vi "Read Roles.vi"(8 "error in (no error)":errorcluster, 11 "EnemyPossessionAtOurFieldPlay in":refnum<class "EnemyPossessionAtOurFieldPlay.lvclass">) -> (0 "error out":errorcluster, 2 "Roles":T1, 3 "EnemyPossessionAtOurFieldPlay out":refnum<class "EnemyPossessionAtOurFieldPlay.lvclass">)   [LabVIEW 2020, in "EnemyPossessionAtOurFieldPlay.lvclass"]
uses:
  EnemyPossessionAtOurFieldPlay.lvclass
  EnemyPossessionAtOurFieldRoles.ctl
  ShootRole_class/ShootRole.lvclass
  MarkerRole_class/MarkerRole.lvclass
  EnemyPossessionAtOurFieldPlay.lvclass/EnemyPossessionAtOurFieldPlay.ctl
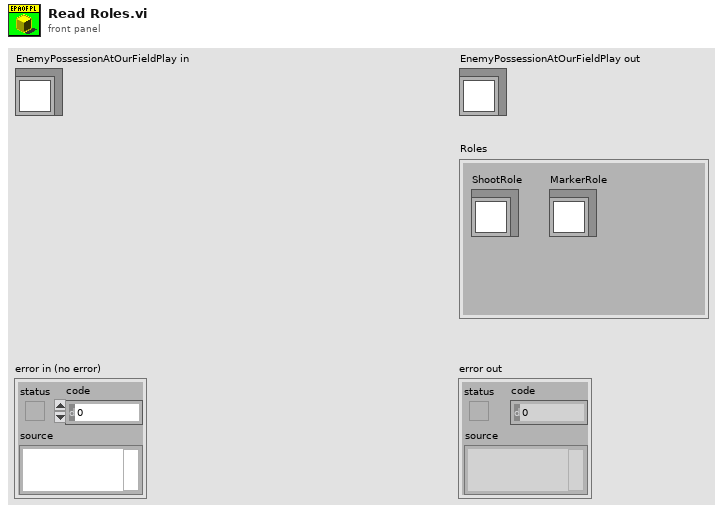
[diagram p1: front panel]
types:
  T1 = typedef "EnemyPossessionAtOurFieldRoles.ctl" = cluster{"ShootRole":refnum<class "ShootRole.lvclass">, "MarkerRole":refnum<class "MarkerRole.lvclass">}
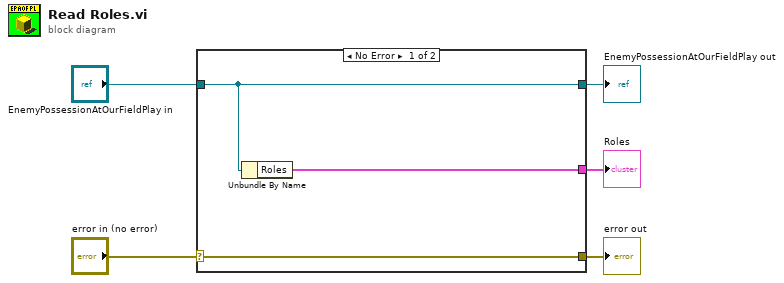
[diagram p0: block diagram]
diagram:
  n1 = case shown="No Error" "error in (no error)" {
    selector: "error in (no error)" -> [w8 w9]
    tunnel: [w8 w9] -> w4
    tunnel: [w7 w10] -> w2
    tunnel: "EnemyPossessionAtOurFieldPlay in" -> [w7 w10]
    tunnel: [w6 _] -> w1
    frame No Error {
      n2 = Unbundle By Name(w7) -> ("Roles"=w6:T1)
    }
    frame Error {
    }
  }
  "error out" <- w4
  "EnemyPossessionAtOurFieldPlay out" <- w2
  "Roles" <- w1
